vi "Actor Core.vi"(8 "error in":errorcluster, 11 "Configuration UI in":refnum<class "Configuration UI.lvclass">) -> (0 "error out":errorcluster, 3 "Actor out":refnum<class "Actor.lvclass">)   [LabVIEW 2019, in "Configuration UI.lvlib" / "Configuration UI.lvclass"]
doc: "This is the user interface panel to edit the config.ini file."
uses:
  Project/Configuration UI.lvclass
  C:/Users/Public/Documents/Development/builds/Engine/Engine.lvlibp/Project/Engine.lvclass
  builds/Engine/Actor Framework.lvlibp/1abvi3w/vi.lib/ActorFramework/Actor/Actor.lvclass
  Project/Configuration UI.lvclass/Configuration UI.ctl
  Configuration UI Messages/Select Instrument Msg/Select Instrument Msg.lvclass/Select Instrument Msg.ctl
  Accessors/Write Instrument Listbox.vi
  Accessors/Write Keys Refnum.vi
  Accessors/Write Signal Refnum.vi
  builds/Engine/Engine.lvlibp/Accessors/Read Self Q.vi
  builds/Engine/Actor Framework.lvlibp/1abvi3w/vi.lib/ActorFramework/Message Enqueuer/Enqueue.vi
  builds/Engine/Actor Framework.lvlibp/1abvi3w/vi.lib/ActorFramework/Message Enqueuer/Message Enqueuer.lvclass
  Configuration UI Messages/Add Device Msg/Add Device Msg.lvclass
  Configuration UI Messages/Reset Msg/Reset Msg.lvclass
  Configuration UI Messages/Select Instrument Msg/Select Instrument Msg.lvclass
  Configuration UI Messages/Remove Device Msg/Remove Device Msg.lvclass
  Configuration UI Messages/Save Keys Msg/Save Keys Msg.lvclass
  builds/Base Software/Panels/Prime Panel.lvlibp/Project/Prime Panel.lvclass
  builds/Engine/Panel Manager.lvlibp/Panel Actor/Panel Actor.lvclass
  C:/Users/Public/Documents/Development/builds/Engine/Panel Manager.lvlibp/Panel Actor/Panel Actor.lvclass
panel:
  in  "Remove Button":bool
  in  "Add Button":bool
  in  "Instruments":i32(listbox)
  in  "Cancel Button":bool
  in  "Save Button":bool
  in  "Keys":i32(listbox)
  out "Signal List":i32(listbox)
  # "Key"
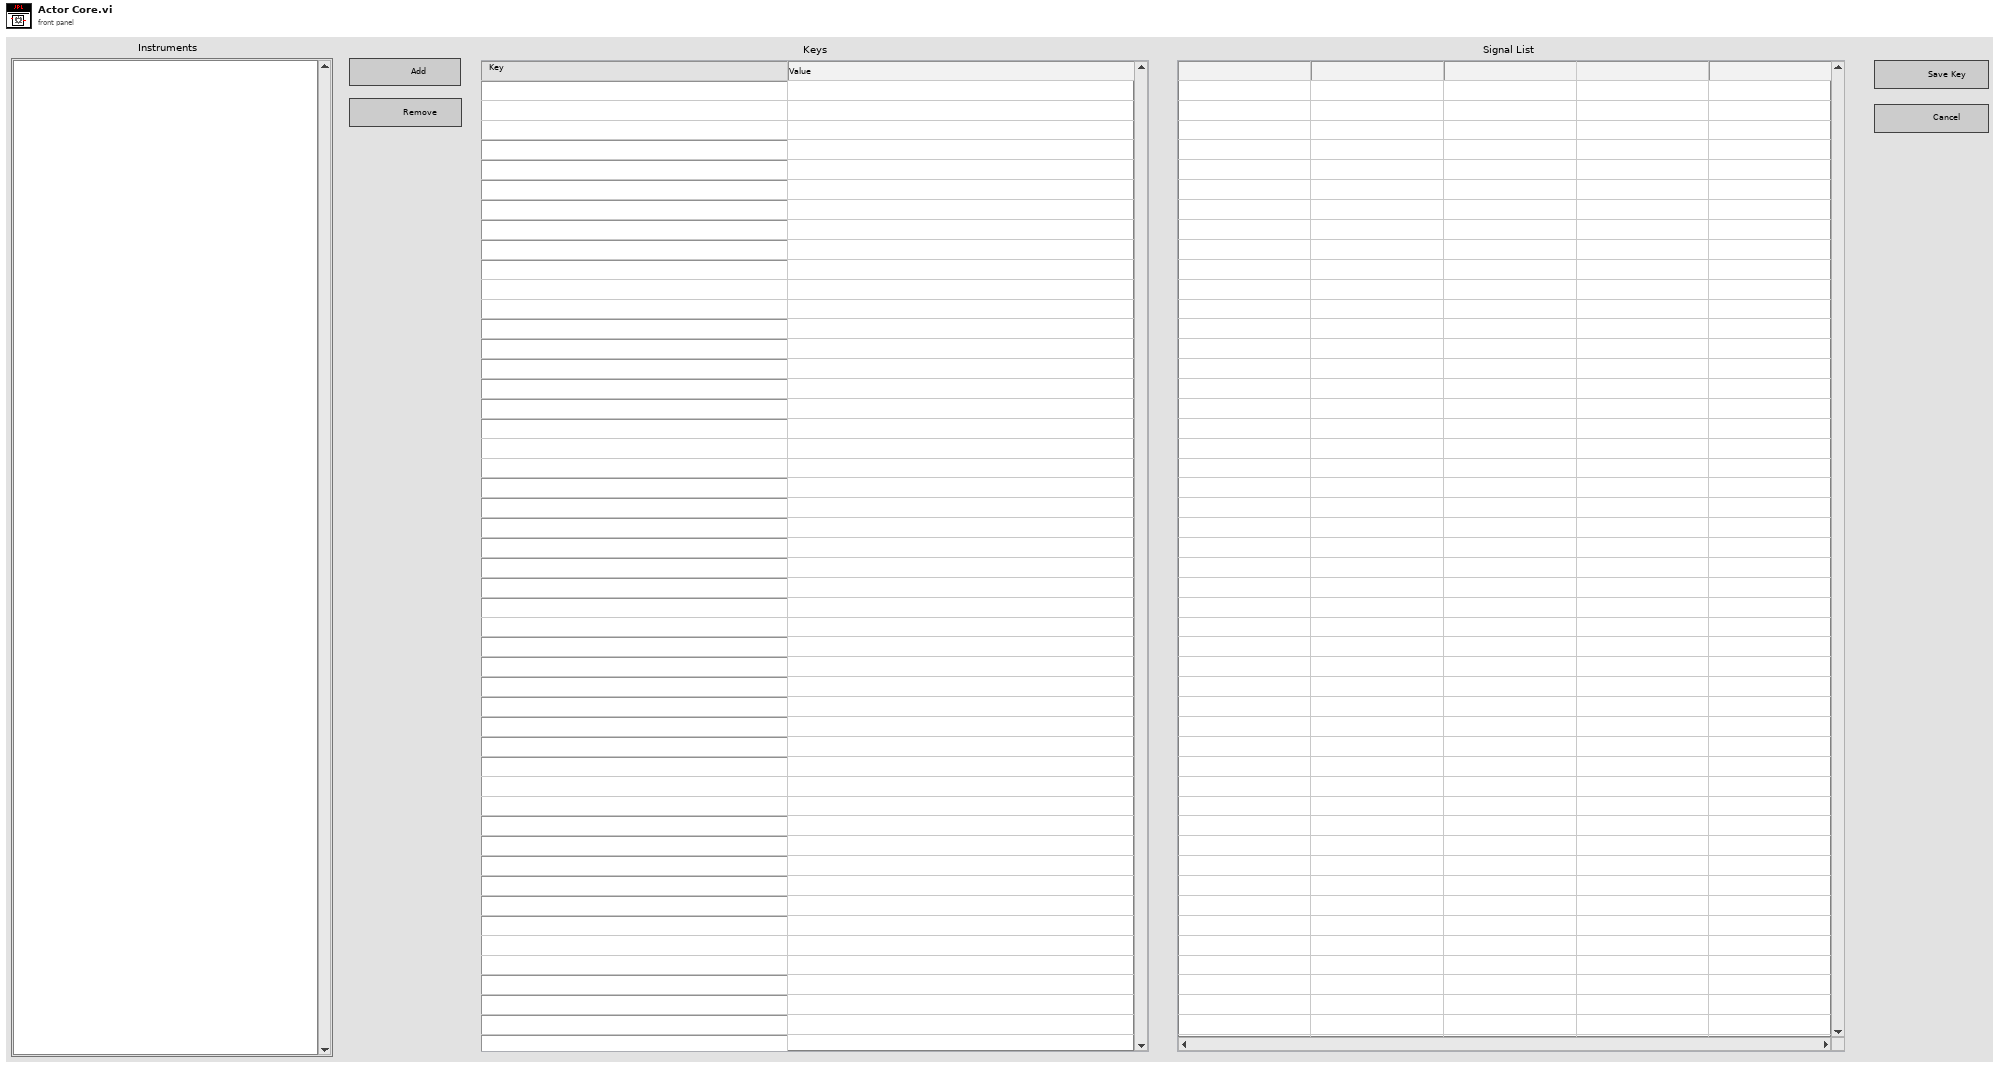
[diagram p1: front panel]
types:
  T1 = typedef "LVPoint32TypeDef.ctl" = cluster{"Horizontal":i32, "Vertical":i32}
  T2 = typedef "LVRowAndColumnTypeDef.ctl" = cluster{"Row":i32, "Column":i32}
  T3 = typedef "eventvkey.ctl" = enum16{"ASCII", "Enter", "Return", "Shift", "Ctrl", "Alt", "Cmd", "Opt", "Caps", "NumLock", "Clear", "Break", "Up", "Down", "Left", "Right", "Insert", "Delete", "Home", "End", "PageUp", "PageDown", "Escape", "Help", "Pause", "ScrollLock", "F1", "F2", "F3", "F4", "F5", "F6", "F7", "F8", "F9", "F10", "F11", "F12", "F13", "F14", "F15", "F16", "F17", "F18", "F19", "F20", "F21", "F22", "F23", "F24", "Play", "VolumeUp", "VolumeDown", "Mute", "Two Byte Char"}
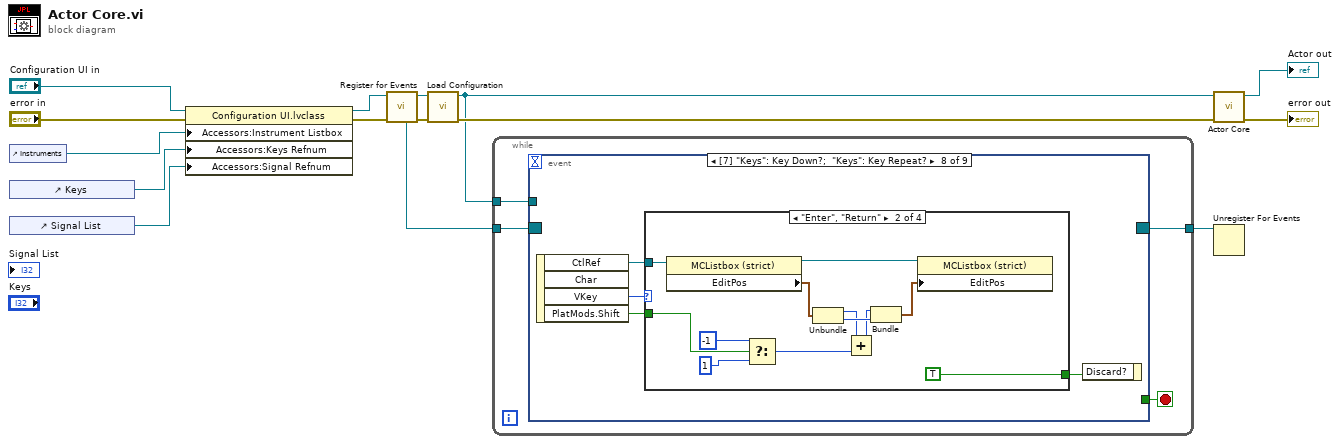
[diagram p0: block diagram]
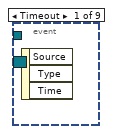
[diagram p2: hidden frame]
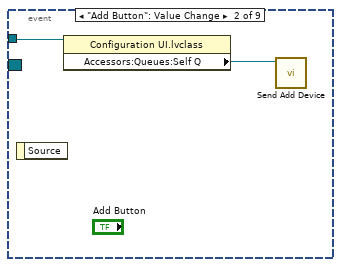
[diagram p3: hidden frame]
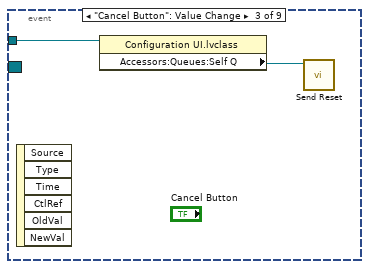
[diagram p4: hidden frame]
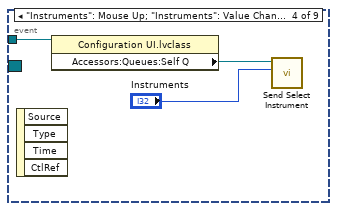
[diagram p5: hidden frame]
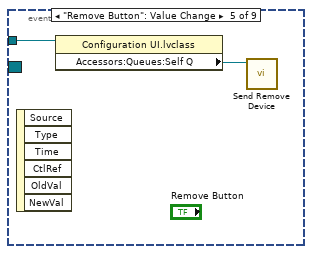
[diagram p6: hidden frame]
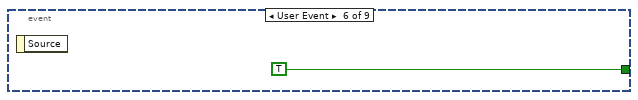
[diagram p7: hidden frame]
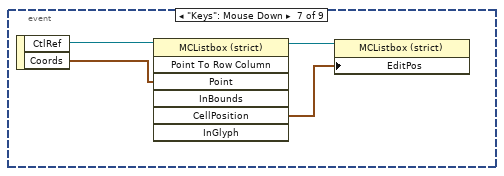
[diagram p8: hidden frame]
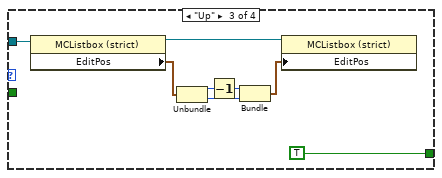
[diagram p10: hidden frame]
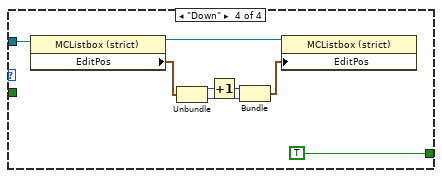
[diagram p11: hidden frame]
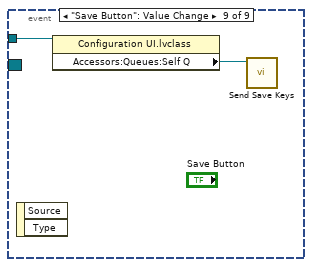
[diagram p12: hidden frame]
diagram:
  n1 = control-ref of="Instruments"() -> (w14:refnum<vi>)
  n2 = control-ref of="Keys"() -> (w13:refnum<vi>)
  n3 = control-ref of="Signal List"() -> (w12:refnum<vi>)
  n4 = property class="Configuration UI.lvclass"(reference="Configuration UI in", error in="error in", "Accessors:Instrument Listbox"=w14, "Accessors:Keys Refnum"=w13, "Accessors:Signal Refnum"=w12) -> (reference out=w11:refnum<class "Configuration UI.lvclass">, error out=w10:errorcluster)
  n5 = call "Register for Events.vi"("Error In"=w10, "Panel Actor in"=w11) -> ("Error Out"=w8:errorcluster, "Panel Actor out"=w9:refnum<class "Configuration UI.lvclass">, "Pnl Actor"=w3:refnum<event-registration>)  [unwired: 6 in, 1 out]
  n6 = call "Load Configuration.vi"("error in"=w8, "Configuration UI in"=w9) -> ("error out"=w7:errorcluster, "Configuration UI out"=w2:refnum<class "Configuration UI.lvclass">)  [unwired: 8 in]
  n7 = while {
    tunnel: w3 -> [w19]
    tunnel: [w17] -> w1
    tunnel: w2 -> [w18]
    stop <- w16 stop-if-true
    n8 = event shown="[7] \"Keys\": Key Down?;  \"Keys\": Key Repeat?" {
      selector: w19 -> [_ _ _ _ _ _ _ _ _]
      dyn-events: [_ _ _ _ _ _ _ _ _] -> w17
      timeout: _ -> [_ _ _ _ _ _ _ _ _]
      tunnel: w18 -> [_ w21 w23 w26 w28 _ _ _ w67]
      tunnel: [_ _ _ _ _ TRUE _ _ _] -> w16
      event Timeout {
        n9 = event-data() -> ()  [unwired: 1 in, 3 out]
      }
      event "Add Button": Value Change {
        n10 = event-data() -> ()  [unwired: 1 in, 1 out]
        n11 = property class="Configuration UI.lvclass"(reference=w21) -> ("Accessors:Queues:Self Q"=w20:refnum<class "Message Enqueuer.lvclass">)  [unwired: 1 in, 2 out]
        n12 = call "Send Add Device.vi"("Message Enqueuer"=w20) -> ()  [unwired: 9 in, 2 out]
      }
      event "Cancel Button": Value Change {
        n13 = event-data() -> ()  [unwired: 1 in, 6 out]
        n14 = property class="Configuration UI.lvclass"(reference=w23) -> ("Accessors:Queues:Self Q"=w22:refnum<class "Message Enqueuer.lvclass">)  [unwired: 1 in, 2 out]
        n15 = call "Send Reset.vi"("Message Enqueuer"=w22) -> ()  [unwired: 9 in, 2 out]
      }
      event "Instruments": Mouse Up; "Instruments": Value Change {
        n16 = event-data() -> ()  [unwired: 1 in, 4 out]
        n17 = property class="Configuration UI.lvclass"(reference=w26) -> ("Accessors:Queues:Self Q"=w25:refnum<class "Message Enqueuer.lvclass">)  [unwired: 1 in, 2 out]
        n18 = call "Send Select Instrument.vi"("Selected"="Instruments", "Message Enqueuer"=w25) -> ()  [unwired: 8 in, 2 out]
      }
      event "Remove Button": Value Change {
        n19 = event-data() -> ()  [unwired: 1 in, 6 out]
        n20 = property class="Configuration UI.lvclass"(reference=w28) -> ("Accessors:Queues:Self Q"=w27:refnum<class "Message Enqueuer.lvclass">)  [unwired: 1 in, 2 out]
        n21 = call "Send Remove Device.vi"("Message Enqueuer"=w27) -> ()  [unwired: 9 in, 2 out]
      }
      event User Event {
        n22 = event-data() -> ()  [unwired: 1 in, 1 out]
      }
      event "Keys": Mouse Down {
        n23 = event-data() -> ("CtlRef"=w33:refnum<vi>, "Coords"=w32:T1)  [unwired: 1 in]
        n24 = invoke class="MCListbox (strict)" method="Point To Row Column"(reference=w33, "Point"=w32) -> (reference out=w31:refnum<vi>, "CellPosition"=w30:T2)  [unwired: 5 in, 5 out]
        n25 = property class="MCListbox (strict)"(reference=w31, "EditPos"=w30) -> ()  [unwired: 1 in, 2 out]
      }
      event "Keys": Key Down?; "Keys": event type 3.0.x8000000b {
        n26 = event-data() -> ("CtlRef"=w35:refnum<vi>, "VKey"=w37:T3, "PlatMods.Shift"=w34:bool)  [unwired: 1 in, 1 out]
        n27 = case shown="\"Enter\", \"Return\"" w37 {
          tunnel: [_ TRUE TRUE TRUE] -> w36
          tunnel: w35 -> [_ w48 w56 w64]
          tunnel: w34 -> [_ w40 _ _]
          frame "ASCII", Default {
          }
          frame "Enter", "Return" {
            n28 = property class="MCListbox (strict)"(reference=w48) -> (reference out=w47:refnum<vi>, "EditPos"=w46:T2)  [unwired: 1 in, 1 out]
            n29 = Select(t=-1, s=w40, f=1) -> (s? t:f=w38:i32)
            n30 = Unbundle(w46) -> ("Row"=w43:i32, "Column"=w45:i32)
            n31 = Add(x=w43, y=w38) -> (x+y=w42:i32)
            n32 = Bundle(w42, "Column"=w45) -> (w44:cluster{i32, "Column":i32})  [unwired: 1 in]
            n33 = property class="MCListbox (strict)"(reference=w47, "EditPos"=w44) -> ()  [unwired: 1 in, 2 out]
          }
          frame "Up" {
            n34 = property class="MCListbox (strict)"(reference=w56) -> (reference out=w55:refnum<vi>, "EditPos"=w54:T2)  [unwired: 1 in, 1 out]
            n35 = Unbundle(w54) -> ("Row"=w51:i32, "Column"=w53:i32)
            n36 = Decrement(x=w51) -> (x-1=w50:i32)
            n37 = Bundle(w50, "Column"=w53) -> (w52:cluster{i32, "Column":i32})  [unwired: 1 in]
            n38 = property class="MCListbox (strict)"(reference=w55, "EditPos"=w52) -> ()  [unwired: 1 in, 2 out]
          }
          frame "Down" {
            n39 = property class="MCListbox (strict)"(reference=w64) -> (reference out=w63:refnum<vi>, "EditPos"=w62:T2)  [unwired: 1 in, 1 out]
            n40 = Unbundle(w62) -> ("Row"=w59:i32, "Column"=w61:i32)
            n41 = Increment(x=w59) -> (x+1=w58:i32)
            n42 = Bundle(w58, "Column"=w61) -> (w60:cluster{i32, "Column":i32})  [unwired: 1 in]
            n43 = property class="MCListbox (strict)"(reference=w63, "EditPos"=w60) -> ()  [unwired: 1 in, 2 out]
          }
        }
        n44 = event-data("Discard?"=w36) -> ()  [unwired: 1 in, 1 out]
      }
      event "Save Button": Value Change {
        n45 = event-data() -> ()  [unwired: 1 in, 2 out]
        n46 = property class="Configuration UI.lvclass"(reference=w67) -> ("Accessors:Queues:Self Q"=w66:refnum<class "Message Enqueuer.lvclass">)  [unwired: 1 in, 2 out]
        n47 = call "Send Save Keys.vi"("Message Enqueuer"=w66) -> ()  [unwired: 9 in, 2 out]
      }
    }
  }
  n48 = call-parent "Actor Core.vi"("error in"=w7, "Prime Panel in"=w2) -> ("error out"=→"error out":errorcluster, "Actor out"=→"Actor out":refnum<class "Actor.lvclass">)  [unwired: 8 in]
  n49 = Unregister For Events(event registration refnum=w1) -> ()  [unwired: 1 in, 1 out]
